vi "Associate Instruments to Paths.vi"(0 "Vector Abstract Path Group in":refnum<class "Vector Abstract Path Group.lvclass">, 5 "TSM Context":T1, 11 "error in (no error)":errorcluster) -> (4 "Vector Abstract Path Group out":refnum<class "Vector Abstract Path Group.lvclass">, 15 "error out":errorcluster)   [LabVIEW 2023, in "RFFixtureCharact.Public.lvlib" / "Vector Abstract Path Group.lvclass"]
uses:
  <vilib>/NI_TestStand_SemiconductorModule/NI_TestStand_Semiconductor_Module.lvlibp/PinMap/General/SemiconductorModuleContext.ctl
  Vector Abstract Path Group.lvclass
  Vector Abstract Path Group.lvclass/Vector Abstract Path Group.ctl
  <vilib>/NI_TestStand_SemiconductorModule/NI_TestStand_Semiconductor_Module.lvlibp
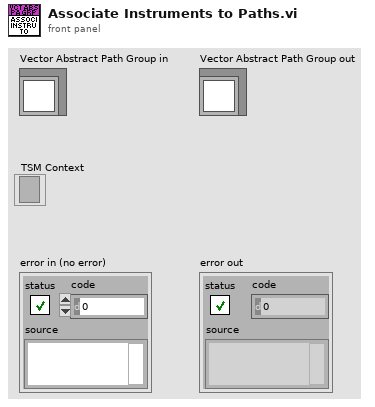
[diagram p1: front panel]
types:
  T1 = typedef "NI_TestStand_Semiconductor_Module.lvlibp/SemiconductorModuleContext.ctl" = refnum<k7>
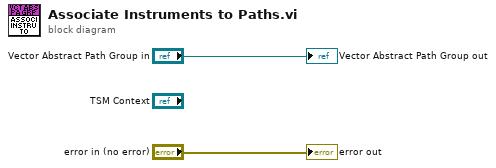
[diagram p0: block diagram]
diagram:
  "error out" <- "error in (no error)"
  "Vector Abstract Path Group out" <- "Vector Abstract Path Group in"
